vi "Max-Min Decimation.vi"(6 "Which graph?":enum16{"Main graph", "Timeline graph"}(ring)=enum."Timeline graph", 9 "Data.Y-Axis values":sgl[](array[numeric]), 11 "Data.X-Axis values":sgl[](array[numeric]) format="%#_6f") -> (1 "Data.Y-Axis values":sgl[](array[numeric]), 3 "Data.X-Axis values":sgl[](array[numeric]) format="%#_6f")   [LabVIEW 2020]
uses:
  xcontrol/Globals/gl_X-Grapher refs.vi
panel:
  out "dt out":sgl format="%#_6f"
  out "dt in":sgl format="%#_6f"
  out "Plot Area Width (pixels)":u32
  out "Post-Decimation Data Points":i32
  out "Pre-Decimation Data Points":i32
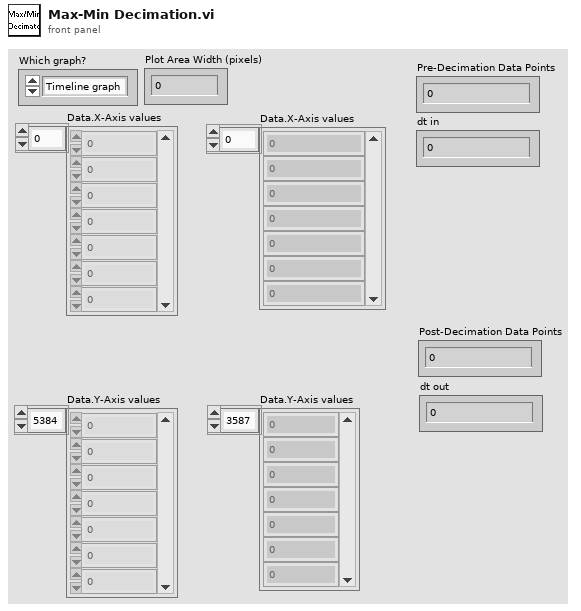
[diagram p1: front panel]
types:
  T1 = typedef "XGrapher.xctl/Xctrl-Waveform graph ref.ctl" = refnum<vi>
  T2 = typedef "XGrapher.xctl/Xctrl-Timeline graph ref.ctl" = refnum<vi>
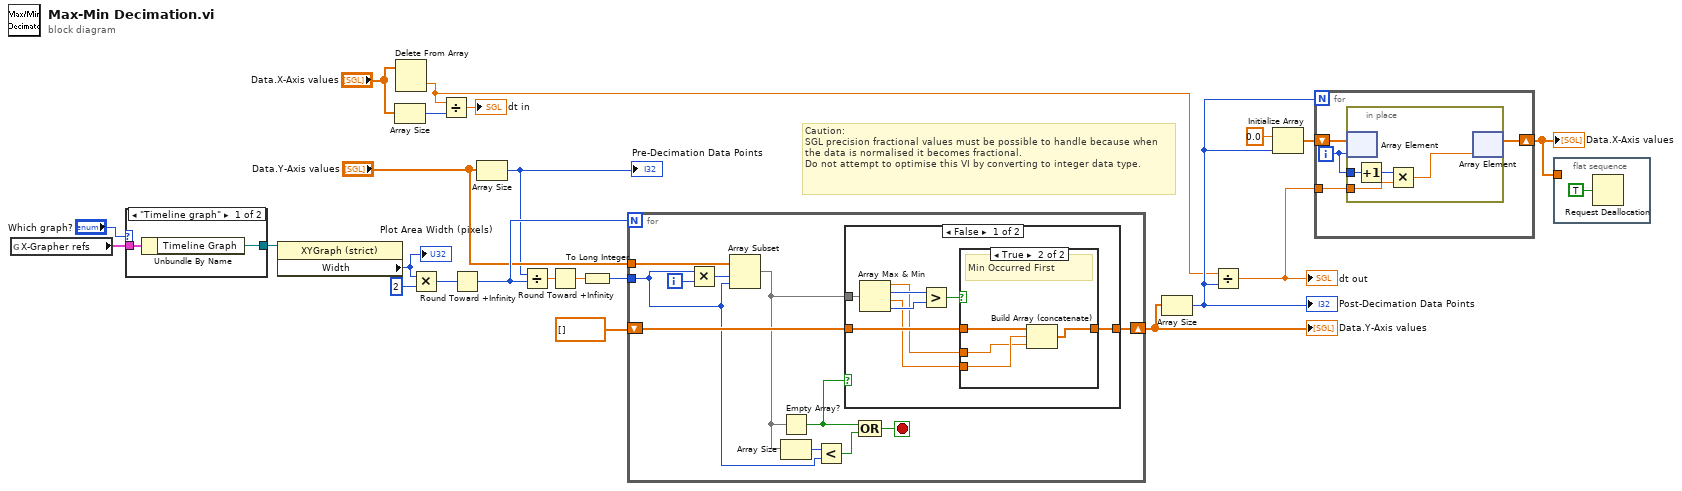
[diagram p0: block diagram]
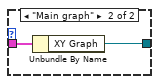
[diagram p2: hidden frame]
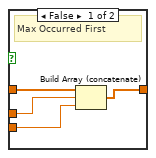
[diagram p3: hidden frame]
diagram:
  # "Caution:\nSGL precision fractional values must be possible to handle because when the data is normalised it becomes fractional.\nDo not attempt to optimise this VI by converting to integer data type."
  n1 = global read "gl_X-Grapher refs.vi" "X-Grapher refs"() -> (w17:cluster{"XY Graph":T1, "Timeline Graph":T2})
  n2 = case shown="\"Timeline graph\"" "Which graph?" {
    tunnel: w17 -> [w25 w27]
    tunnel: [w24 w26] -> w15
    frame "Timeline graph" {
      n3 = Unbundle By Name(w25) -> ("Timeline Graph"=w24:T2)
    }
    frame "Main graph" {
      n4 = Unbundle By Name(w27) -> ("XY Graph"=w26:T1)
    }
  }
  n5 = property on="Property Node" class="XYGraph (strict)"(reference=w15) -> ("Width"=w14:u32)  [unwired: 1 in, 2 out]
  "Plot Area Width (pixels)" <- w14
  n6 = Array Size(array="Data.X-Axis values") -> (size(s)=w11:i32)
  n7 = Delete From Array(array="Data.X-Axis values") -> (deleted portion=w3:sgl)  [unwired: 2 in, 1 out]
  n8 = Multiply(x=w14, y=u32 2) -> (x*y=w22:u32)
  n9 = Divide(x=w3, y=w11) -> (x/y=→"dt in":sgl)
  n10 = Round Toward +Infinity(x=w22) -> (ceil(x): smallest int >= x=w20:u32)
  n11 = Array Size(array="Data.Y-Axis values") -> (size(s)=w6:i32)
  "Pre-Decimation Data Points" <- w6
  n12 = Divide(x=w6, y=w20) -> (x/y=w18:dbl)
  n13 = Round Toward +Infinity(x=w18) -> (ceil(x): smallest int >= x=w19:dbl)
  n14 = To Long Integer(number=w19) -> (32bit integer=w2:i32)
  n15 = for {
    N: w20 -> [_]
    tunnel: "Data.Y-Axis values" -> [w38]
    tunnel: w2 -> [w31]
    shift-right: [w34] -> w7
    shift-left: sgl[] [] -> [w35]
    i -> [w36]
    stop <- w29 stop-if-true
    n16 = Multiply(x=w31, y=w36) -> (x*y=w37:i32)
    n17 = Array Subset(array=w38, index=w37, length=w31) -> (w33:sgl[])
    n18 = Empty Array?(array=w33) -> (empty?=w28:bool)
    n19 = Array Size(array=w33) -> (size(s)=w32:i32)
    n20 = Less?(x=w32, y=w31) -> (x < y?=w30:bool)
    n21 = case shown="False" w28 {
      tunnel: w35 -> [w43 w55]
      tunnel: [w40 w55] -> w34
      tunnel: w33 -> [w39 _]
      frame False {
        n22 = Array Max & Min(array=w39) -> (max value=w41:sgl, max index (indices)=w46:i32, min value=w42:sgl, min index (indices)=w45:i32)
        n23 = Greater?(x=w46, y=w45) -> (0:w44:bool)
        n24 = case shown="True" w44 {
          tunnel: w43 -> [w50 w54]
          tunnel: w42 -> [w48 w53]
          tunnel: w41 -> [w49 w52]
          tunnel: [w47 w51] -> w40
          frame False {
            # "Max Occurred First"
            n25 = Build Array (concatenate)(w50, w49, w48) -> (w47:sgl[])
          }
          frame True {
            # "Min Occurred First"
            n26 = Build Array (concatenate)(w54, w53, w52) -> (w51:sgl[])
          }
        }
      }
      frame True {
      }
    }
    n27 = Compound Arithmetic op=OR(w28, w30) -> (w29:bool)
  }
  "Data.Y-Axis values" <- w7
  n28 = Array Size(array=w7) -> (size(s)=w8:i32)
  "Post-Decimation Data Points" <- w8
  n29 = Divide(x=w3, y=w8) -> (x/y=w5:sgl)
  "dt out" <- w5
  n30 = Initialize Array(sgl 0.0 ("element"), w8) -> (w9:sgl[])
  n31 = for {
    N: w8 -> [_]
    shift-right: [w56] -> w1
    shift-left: w9 -> [w59]
    tunnel: w5 -> [w57]
    i -> [w58]
    n32 = in-place {
      in-place-border: w58 -> [w63]
      in-place-border: w57 -> [w61]
      n33 = in-place-array #1(w59, w58) -> ()  [unwired: 1 out]
      n34 = Increment(x=w63) -> (x+1=w62:i32)
      n35 = Multiply(x=w62, y=w61) -> (x*y=w60:sgl)
      n36 = in-place-array #1(w60) -> (w56:sgl[])  [unwired: 1 out]
    }
  }
  "Data.X-Axis values" <- w1
  n37 = flat-sequence {
    tunnel: w1 -> [_]
    frame #0 {
      n38 = Request Deallocation(TRUE ("flag")) -> ()
    }
  }
